vi "Pump modulator.vi"(2 "y U8 in":dbl) -> (0 "y U8 modulated":u8)   [LabVIEW 2012]
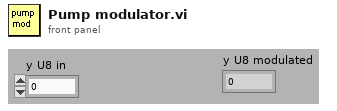
[diagram p1: front panel]
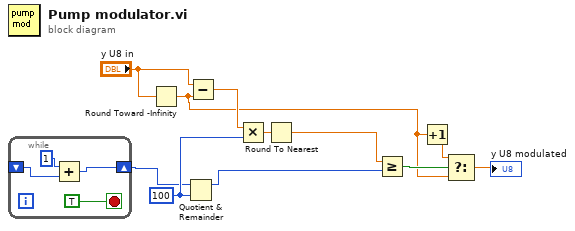
[diagram p0: block diagram]
diagram:
  w9 = 100 ("y")
  n1 = while {
    shift-right: [w13] -> w1
    shift-left: _ -> [w14]
    stop <- TRUE stop-if-true
    n2 = Add(x=1, y=w14) -> (x+y=w13:i32)
  }
  n3 = Round Toward -Infinity(1:"y U8 in") -> (0:w3:dbl)
  n4 = Quotient & Remainder(x=w1, y=w9) -> (x-y*floor(x/y)=w7:i32)  [unwired: 1 out]
  n5 = Subtract(x="y U8 in", y=w3) -> (x-y=w11:dbl)
  n6 = Multiply(x=w11, y=w9) -> (x*y=w10:dbl)
  n7 = Round To Nearest(number=w10) -> (nearest integer value=w8:dbl)
  n8 = Greater Or Equal?(x=w8, y=w7) -> (x >= y?=w6:bool)
  n9 = Increment(x=w3) -> (x+1=w2:dbl)
  n10 = Select(t=w2, s=w6, f=w3) -> (s? t:f=→"y U8 modulated":dbl)
